vi "ReadIMU.vi"() -> ()   [LabVIEW 2015]
doc: "The myRIO Project template acquires acceleration data from the onboard accelerometer and displays the changes of acceleration values in a waveform chart."
uses:
  <vilib>/myRIO/Instrument Drivers/Onboard IO/I2C/typedefs/I2C User Configuration.ctl
  <vilib>/myRIO/Instrument Drivers/Onboard IO/I2C/typedefs/I2C Transfer Rate.ctl
  <vilib>/myRIO/Instrument Drivers/Onboard IO/I2C/typedefs/I2C Reference.ctl
  <vilib>/myRIO/Common/Instrument Driver Framework/Utilities/typedefs/myRIO Generic Hardware Reference.ctl
  <vilib>/myRIO/Common/Instrument Driver Framework/Utilities/typedefs/Hardware Version Enum.ctl
  <vilib>/myRIO/Common/Instrument Driver Framework/Utilities/typedefs/myRIO v1.0 Reference.ctl
  <vilib>/myRIO/Common/Instrument Driver Framework/Utilities/typedefs/Generic FPGA Reference.ctl
  <vilib>/myRIO/Common/Instrument Driver Framework/myRIO v1.0/I2C/typedefs/I2C Channels Enum.ctl
  <vilib>/myRIO/Instrument Drivers/Onboard IO/I2C/typedefs/I2C Configuration.ctl
  <vilib>/userdefined/High Color/nirio_resource_hc.ctl
  <vilib>/myRIO/Common/Instrument Driver Framework/Utilities/vis/Is FPGA Ref Available.vi
  <vilib>/myRIO/Common/Instrument Driver Framework/myRIO v1.0/I2C/vis/myRIO v1.1 Open I2C.vi
  <vilib>/myRIO/Instrument Drivers/Onboard IO/I2C/vis/Configure.vi
  <vilib>/myRIO/Instrument Drivers/Onboard IO/I2C/vis/Write.vi
  <vilib>/myRIO/Common/Instrument Driver Framework/Utilities/vis/Validate Channels.vi
  <vilib>/myRIO/Common/Instrument Driver Framework/myRIO v1.0/I2C/vis/myRIO v1.0 Reserve I2C.vi
  <vilib>/myRIO/Instrument Drivers/Onboard IO/I2C/vis/Read.vi
  <vilib>/myRIO/Common/Instrument Driver Framework/myRIO v1.0/I2C/vis/myRIO v1.0 Build MUX Configuration I2C.vi
  <vilib>/myRIO/Common/Instrument Driver Framework/myRIO v1.0/Resource Manager/vis/myRIO v1.0 Reserve Channel List.vi
  <vilib>/myRIO/Common/Instrument Driver Framework/myRIO v1.0/Resource Manager/vis/myRIO v1.0 Create Configuration List.vi
  <vilib>/myRIO/Common/Instrument Driver Framework/myRIO v1.0/Resource Manager/vis/myRIO v1.0 Reserve Channel.vi
  <vilib>/myRIO/Common/Instrument Driver Framework/myRIO v1.0/Resource Manager/vis/myRIO v1.0 Unreserve Channel.vi
  <vilib>/myRIO/Common/Instrument Driver Framework/myRIO v1.0/Resource Manager/vis/myRIO v1.0 Build Mutex Name.vi
  <vilib>/Utility/VariantDataType/GetNumericInfo.vi
  <vilib>/Utility/error.llb/Error Cluster From Error Code.vi
  <vilib>/myRIO/Common/Instrument Driver Framework/myRIO v1.0/myRIO v1.1 Open.vi
  <vilib>/myRIO/Common/Instrument Driver Framework/Utilities/vis/IO Manager.vi
  <vilib>/myRIO/Common/Instrument Driver Framework/Utilities/vis/Configuration Manager.vi
  <vilib>/myRIO/Common/Instrument Driver Framework/myRIO v1.0/Resource Manager/vis/myRIO v1.0 Configure IO.vi
  <vilib>/myRIO/Common/Instrument Driver Framework/myRIO v1.0/myRIO v1.0 Close.vi
  <vilib>/myRIO/Common/Instrument Driver Framework/myRIO v1.0/I2C/vis/myRIO v1.0 Configure I2C.vi
  <vilib>/myRIO/Common/Instrument Driver Framework/myRIO v1.0/I2C/vis/myRIO v1.0 Write I2C.vi
  <vilib>/myRIO/Instrument Drivers/Onboard IO/I2C/vis/Smart Open.vi
  <vilib>/myRIO/Common/Instrument Driver Framework/myRIO v1.0/I2C/vis/myRIO v1.0 Read I2C.vi
  <vilib>/myRIO/Express VI/Onboard IO/I2C/I2C Express VI.xnode
  <vilib>/myRIO/Instrument Drivers/Onboard IO/I2C/vis/myRIO I2C Open.xnode
  <vilib>/myRIO/Instrument Drivers/Onboard IO/I2C/I2C.lvlib
panel:
  in  "Stop Button":bool
  in  "error in (no error)":errorcluster
  out "error out":errorcluster
  out "Heading Data":T1
  out "Array":u8[](array[numeric]) format="%b"
  out "Numeric":dbl format="%#_13g"
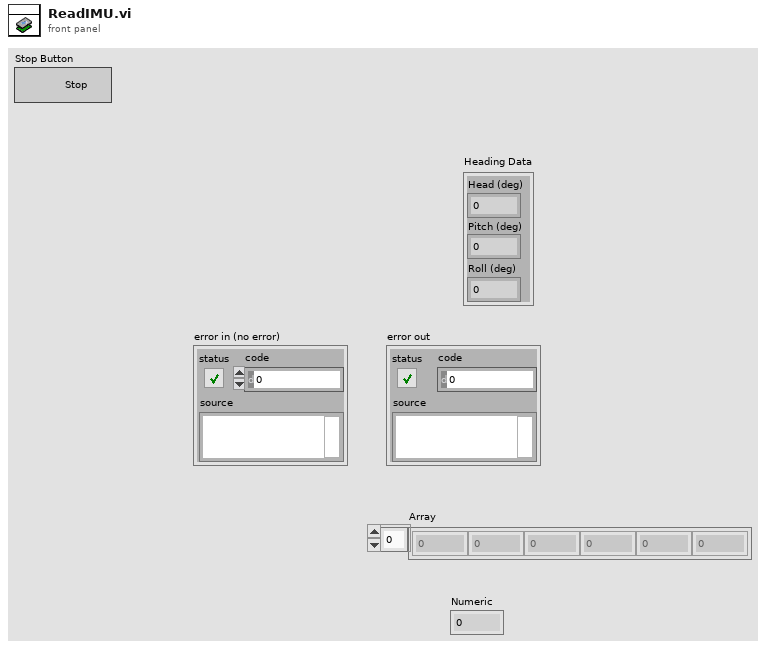
[diagram p1: front panel]
types:
  T1 = cluster{"Head (deg)":dbl, "Pitch (deg)":dbl, "Roll (deg)":dbl}
  T2 = typedef "I2C.lvlib/I2C Reference.ctl" = cluster{"myRIO Reference":T3, "I2C Channels Enum":T7, "I2C Configuration":T8}
  T3 = typedef "myRIO Generic Hardware Reference.ctl" = cluster{"myRIO Model":T4, "myRIO Hardware Reference":T5}
  T4 = typedef "Hardware Version Enum.ctl" = enum16{"Unknown", "myRIO-1900", "myRIO-1950", "roboRIO"}
  T5 = typedef "myRIO v1.0 Reference.ctl" = cluster{"Generic FPGA Reference":T6, "Allow multiple opens":bool}
  T6 = typedef "Generic FPGA Reference.ctl" = refnum<k20>
  T7 = typedef "I2C Channels Enum.ctl" = enum16{"Not Connected", "A/I2C", "B/I2C", "I2C/I2C"}
  T8 = typedef "I2C.lvlib/I2C Configuration.ctl" = cluster{"I2C Transfer Rate":T9}
  T9 = typedef "I2C.lvlib/I2C Transfer Rate.ctl" = enum16{"Standard mode (100 kbps)", "Fast mode (400 kbps)"}
  T10 = typedef "I2C.lvlib/I2C User Configuration.ctl" = cluster{"I2C Transfer Rate":T9}
  T11 = typedef "nirio_resource_hc.ctl" = tag
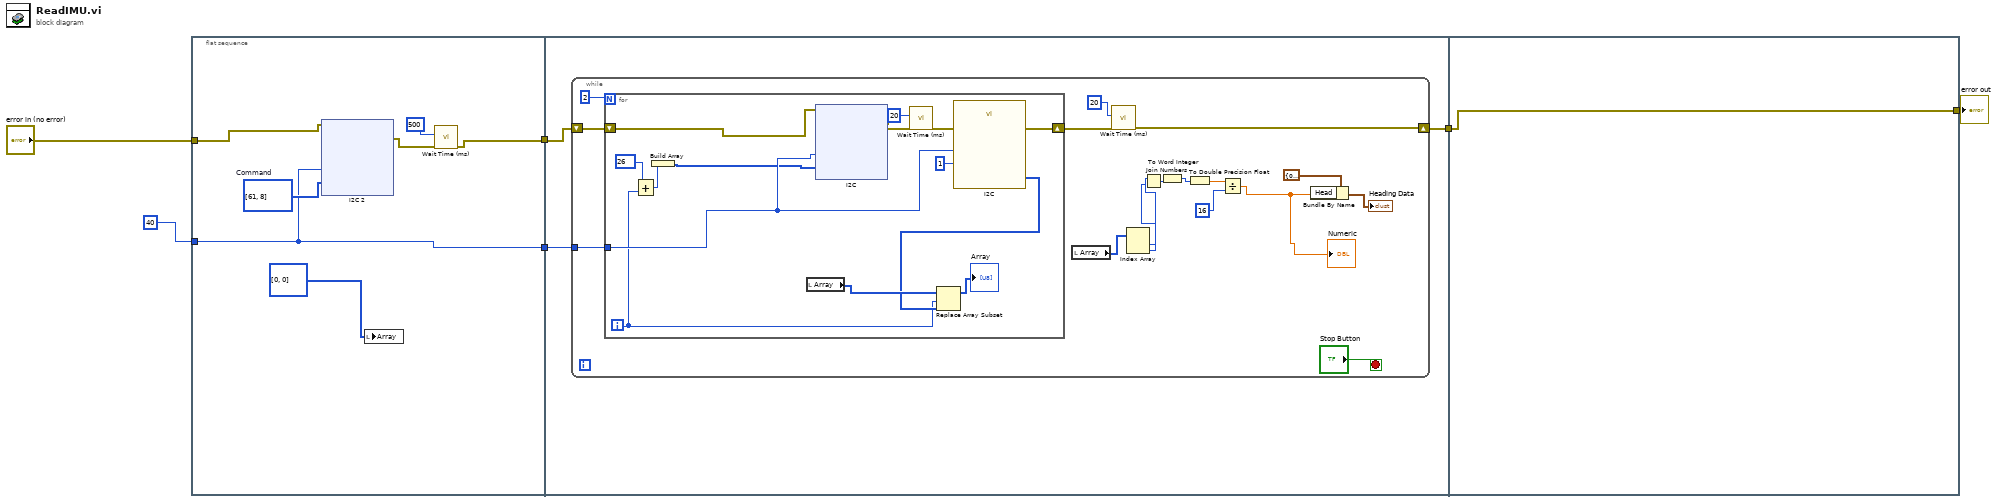
[diagram p0: block diagram]
diagram:
  n1 = flat-sequence {
    tunnel: "error in (no error)" -> [w11]
    tunnel: [w13] -> w6
    tunnel: [w8] -> w5
    tunnel: u8 40 ("Slave Address (7-bit)") -> [w8]
    tunnel: w6 -> [w53]
    tunnel: w5 -> [w52]
    tunnel: [w54] -> w4
    tunnel: w4 -> [w124]
    tunnel: [w124] -> w2
    frame #0 {
      w9 = u8[] [61, 8]  # Command
      n2 = xnode "I2C 2"("Slave Address (7-bit)"=w8, "Bytes to Write"=w9, "error in (no error)"=w11) -> ("error out"=w10:errorcluster)
      n3 = local write "Array"(i32[] [0, 0]) -> ()
      n4 = call "Wait Time (ms).vi"("error in (no error)"=w10, "Wait Time (ms)"=500) -> ("error out"=w13:errorcluster)  [unwired: 9 in]
    }
    frame #1 {
      n5 = while {
        tunnel: w52 -> [w68]
        shift-right: [w61] -> w54
        shift-left: w53 -> [w69]
        stop <- "Stop Button" stop-if-true
        n6 = for {
          N: 2 -> [_]
          tunnel: w68 -> [w80]
          shift-right: [w79] -> w62
          shift-left: w69 -> [w81]
          i -> [w73]
          n7 = Add(x=26 ("Data Byte (0x0)"), y=w73) -> (x+y=w76:i32)
          n8 = Build Array(w76) -> (w78:i32[])
          n9 = local read "Array"() -> (w75:u8[])
          n10 = xnode "I2C"("Slave Address (7-bit)"=w80, "Bytes to Write"=w78, "error in (no error)"=w81) -> ("error out"=w82:errorcluster)
          n11 = call "Wait Time (ms).vi"("error in (no error)"=w82, "Wait Time (ms)"=u32 20) -> ("error out"=w84:errorcluster)  [unwired: 9 in]
          n12 = call "I2C"("Slave Address (7-bit)"=w80, "Byte Count"=u32 1 ("Bytes to Read"), "error in (no error)"=w84) -> ("Bytes Read"=w74:u8[], "error out"=w79:errorcluster)  [unwired: 23 in]
          n13 = Replace Array Subset(array=w75, new element=w74, index=w73) -> (→"Array":u8[])
        }
        n14 = local read "Array"() -> (w59:u8[])
        n15 = call "Wait Time (ms).vi"("error in (no error)"=w62, "Wait Time (ms)"=20) -> ("error out"=w61:errorcluster)  [unwired: 9 in]
        n16 = Index Array(array=w59) -> (element #1=w57:u8, element #2=w58:u8)  [unwired: 2 in]
        n17 = Join Numbers(hi=w58, lo=w57) -> ((hi.lo)=w63:u16)
        n18 = To Word Integer(number=w63) -> (16bit integer=w64:i16)
        n19 = To Double Precision Float(number=w64) -> (double precision float=w67:dbl)
        n20 = Divide(x=w67, y=16) -> (x/y=w56:dbl)
        "Numeric" <- w56
        n21 = Bundle By Name(cluster=cluster{"Head":dbl, "Pitch":dbl, "Roll":dbl} {"Head"=0.0, "Pitch"=0.0, "Roll"=0.0} ("Heading Data"), "Head"=w56) -> (→"Heading Data":cluster{"Head":dbl, "Pitch":dbl, "Roll":dbl})
      }
    }
    frame #2 {
    }
  }
  "error out" <- w2
